vi "Servo_test.vi"() -> ()   [LabVIEW 2009]
doc: "Test function for verifying that the camera servos works as they should. Nothing else needs to be called before."
uses:
  FPGA.lvlib
  Servo.lvlib
panel:
  in  "Pitch":dbl(slide) min=-45.0 max=45.0 scale=-60.0..60.0
  in  "Yaw":dbl(slide) min=-45.0 max=45.0 scale=-45.0..45.0
  in  "stop":bool
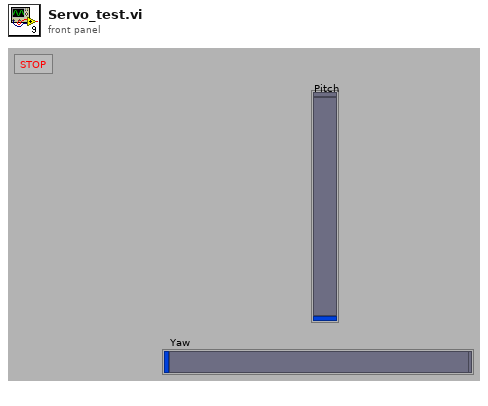
[diagram p1: front panel]
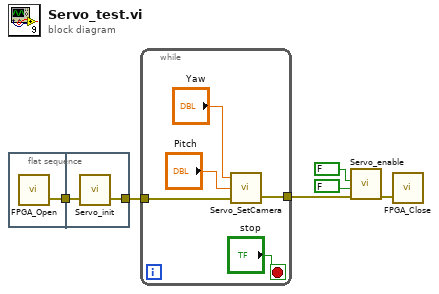
[diagram p0: block diagram]
diagram:
  n1 = flat-sequence {
    tunnel: [w7] -> w1
    tunnel: [w8] -> w6
    tunnel: w1 -> [w9]
    frame #0 {
      n2 = call "FPGA_Open.vi"() -> ("error out"=w7:errorcluster)  [unwired: 3 in]
    }
    frame #1 {
      n3 = call "Servo_init.vi"("error in (no error)"=w9) -> ("error out"=w8:errorcluster)  [unwired: 2 in]
    }
  }
  n4 = while {
    tunnel: w6 -> [w11]
    tunnel: [w10] -> w3
    stop <- "stop" stop-if-true
    n5 = call "Servo_SetCamera.vi"("error in"=w11, "PWM10 Angle in"="Pitch", "PWM9 Angle in"="Yaw") -> ("error out"=w10:errorcluster)  [unwired: 1 in]
  }
  n6 = call "Servo_enable.vi"("error in"=w3, "Set PWM9"=FALSE ("Enable 2"), "Set PWM10"=FALSE ("Enable")) -> ("error out"=w2:errorcluster)  [unwired: 8 in]
  n7 = call "FPGA_Close.vi"("error in (no error)"=w2) -> ()  [unwired: 2 in, 1 out]
